vi "run VI asynchronously.vi"(9 "results reporter":refnum<class "results reporter.lvclass">, 10 "parameters":variant, 11 "VI in":T1) -> ()   [LabVIEW 2014]
uses:
  standard action/call by reference action/function definition.ctl
  results reporter/results reporter.lvclass
  standard action/call by reference action/call function by reference.lvclass
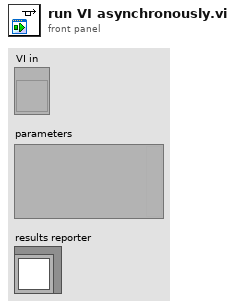
[diagram p1: front panel]
types:
  T1 = typedef "call function by reference.lvclass/function definition.ctl" = refnum<vi>
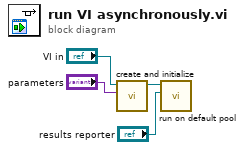
[diagram p0: block diagram]
diagram:
  n1 = call "create and initialize.vi"("parameters"="parameters", "function"="VI in") -> ("call by reference action"=w2:refnum<class "call function by reference.lvclass">)  [unwired: 8 in, 1 out]
  n2 = call "run on default pool.vi"("results reporter"="results reporter", "task"=w2) -> ()  [unwired: 9 in, 1 out]
